vi "LedControl (SubVI).vi"(8 "error in (no error)":errorcluster, 10 "Red/Green [T/F]":bool, 11 "LedRef":refnum<class "Digital Output.lvclass">[](array[class])) -> (0 "error out":errorcluster, 3 "LedRef":refnum<class "Digital Output.lvclass">[](array[class]))   [LabVIEW 2020]
uses:
  <vilib>/CISH Robotics/L4VMX VMXpi/Digital Output/Digital Output.lvclass
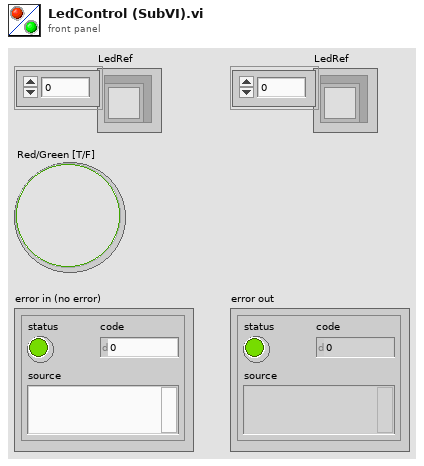
[diagram p1: front panel]
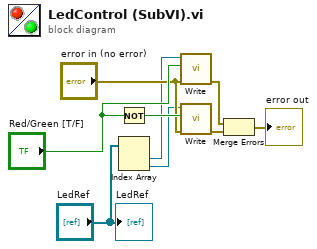
[diagram p0: block diagram]
diagram:
  n1 = Not(x="Red/Green [T/F]") -> (.not. x?=w9:bool)
  n2 = Index Array(array="LedRef") -> (element #1=w4:refnum<class "Digital Output.lvclass">, element #2=w5:refnum<class "Digital Output.lvclass">)  [unwired: 2 in]
  n3 = call <vilib>:"Write.vi"("Error In"="error in (no error)", "Value"="Red/Green [T/F]", "Digital Output Object"=w4) -> ("Error Out"=w2:errorcluster)  [unwired: 7 in, 1 out]
  n4 = call <vilib>:"Write.vi"("Error In"="error in (no error)", "Value"=w9, "Digital Output Object"=w5) -> ("Error Out"=w3:errorcluster)  [unwired: 7 in, 1 out]
  n5 = Merge Errors(w2, w3) -> (→"error out":errorcluster)
  "LedRef" <- "LedRef"
